vi "FFT - Compute dB Level - Single value.vi"(1 "RMS EU Value":dbl, 3 "Unit":string, 7 "Spectrum Display Options":T1) -> (15 "dB Value":dbl)   [LabVIEW 2022 SP3, in "GSwFormDSP.lvclass"]
uses:
  GSwFormDSP.lvclass
  Spectrum Display Options.ctl
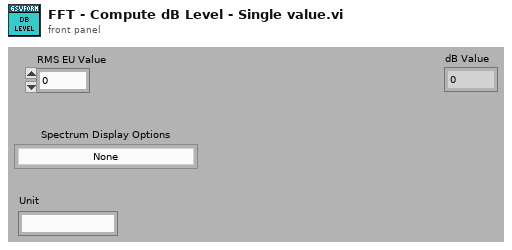
[diagram p1: front panel]
types:
  T1 = typedef "GSwFormDSP.lvclass/Spectrum Display Options.ctl" = enum16{"None", "dB - NO reference value", "dB - Automatic reference value", "dB - Sound SPL (ref 20E-6 Pa)", "dB - Acceleration (ref 1E-6 m/s²)", "dB - Velocity (ref 1E-9 m/s)", "dB - Displacement (ref 1E-12 m)"}
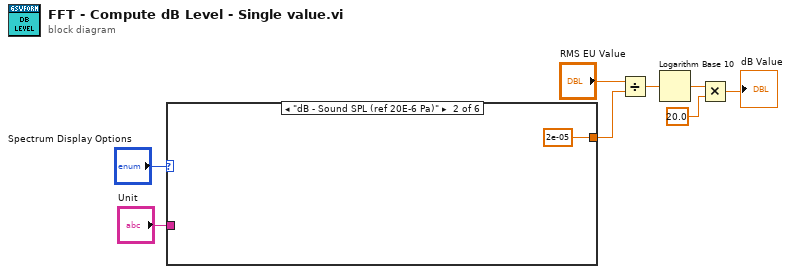
[diagram p0: block diagram]
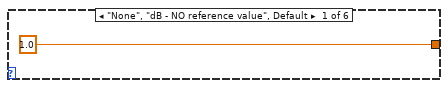
[diagram p2: hidden frame]
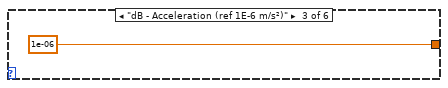
[diagram p3: hidden frame]
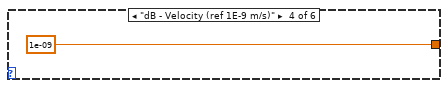
[diagram p4: hidden frame]
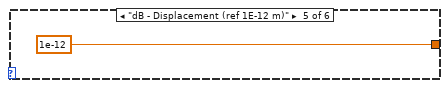
[diagram p5: hidden frame]
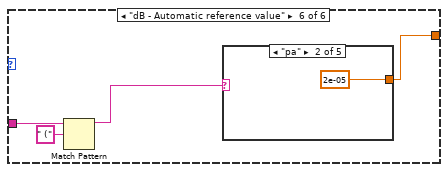
[diagram p6: hidden frame]
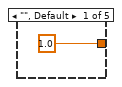
[diagram p7: hidden frame]
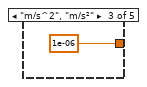
[diagram p8: hidden frame]
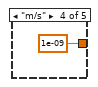
[diagram p9: hidden frame]
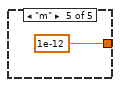
[diagram p10: hidden frame]
diagram:
  n1 = case shown="\"dB - Sound SPL (ref 20E-6 Pa)\"" "Spectrum Display Options" {
    tunnel: [1.0 ("Automatic reference Value") 2e-05 1e-06 1e-09 1e-12 w17] -> w2
    tunnel: "Unit" -> [_ _ _ _ _ w16]
    frame "None", "dB - NO reference value", Default {
    }
    frame "dB - Sound SPL (ref 20E-6 Pa)" {
    }
    frame "dB - Acceleration (ref 1E-6 m/s²)" {
    }
    frame "dB - Velocity (ref 1E-9 m/s)" {
    }
    frame "dB - Displacement (ref 1E-12 m)" {
    }
    frame "dB - Automatic reference value" {
      n2 = Match Pattern(string=w16, regular expression=" (") -> (before substring=w14:string)  [unwired: 1 in, 3 out]
      n3 = case shown="\"pa\"" w14 {
        tunnel: [1.0 2e-05 1e-06 1e-09 1e-12] -> w17
        frame "", Default {
        }
        frame "pa" {
        }
        frame "m/s^2", "m/s²" {
        }
        frame "m/s" {
        }
        frame "m" {
        }
      }
    }
  }
  n4 = Divide(x="RMS EU Value", y=w2) -> (x/y=w7:dbl)
  n5 = Logarithm Base 10(1:w7) -> (0:w5:dbl)
  n6 = Multiply(x=w5, y=20.0) -> (x*y=→"dB Value":dbl)
